vi "QueryROS2.vi"(11 "String":string) -> (3 "Console":string)   [LabVIEW 2022 SP3]
uses:
  Comm_Global.vi
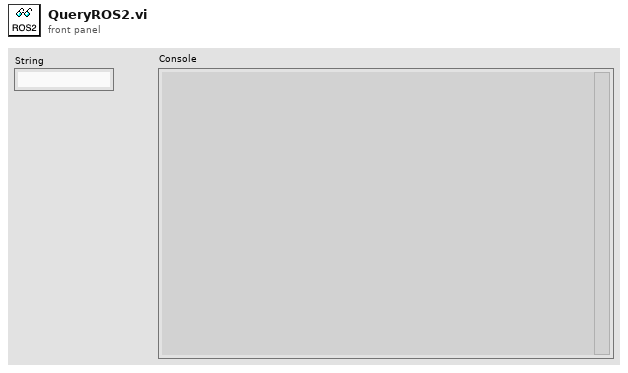
[diagram p1: front panel]
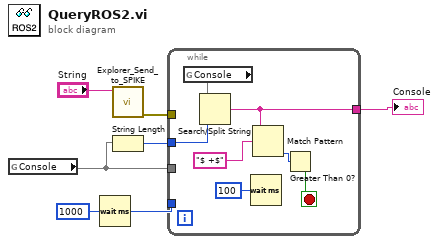
[diagram p0: block diagram]
diagram:
  n1 = global read "Comm_Global.vi" "Console"() -> (w5)
  n2 = Wait (ms)(milliseconds to wait=u32 1000) -> (millisecond timer value=w1:u32)
  n3 = call "Explorer_Send_to_SPIKE.vi"("python"="String") -> ("error out"=w3:errorcluster)  [unwired: 10 in]
  n4 = String Length(string=w5) -> (length=w6:i32)
  n5 = while {
    tunnel: w3 -> [_]
    tunnel: w5 -> [_]
    tunnel: w6 -> [w9]
    tunnel: [w8] -> w7
    tunnel: w1 -> [_]
    stop <- w11 stop-if-true
    n6 = global read "Comm_Global.vi" "Console"() -> (w10)
    n7 = Search/Split String(string=w10, offset (0)=w9) -> (match + rest of string=w8:string)  [unwired: 1 in, 2 out]
    n8 = Wait (ms)(milliseconds to wait=u32 100) -> ()  [unwired: 1 out]
    n9 = Match Pattern(string=w8, regular expression="$ +$") -> (offset past match=w12:i32)  [unwired: 1 in, 3 out]
    n10 = Greater Than 0?(x=w12) -> (x > 0?=w11:bool)
  }
  "Console" <- w7
